vi "GetType.vi"(8 "error in (no error)":errorcluster, 11 "Load Pattern Msg":refnum<class "Load Pattern Msg.lvclass">) -> (0 "error out":errorcluster, 2 "Data Sample":variant, 3 "Load Pattern Msg":refnum<class "Load Pattern Msg.lvclass">)   [LabVIEW 2016, in "CS++PPG.lvlib" / "Load Pattern Msg.lvclass"]
uses:
  Load Pattern Msg.lvclass
  Load Pattern Msg.lvclass/Load Pattern Msg.ctl
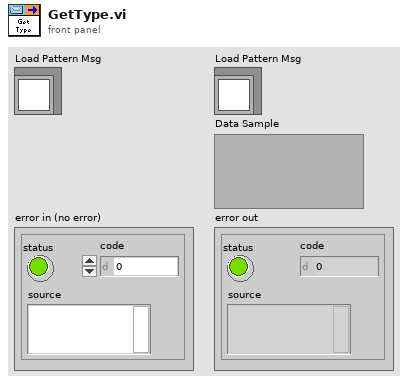
[diagram p1: front panel]
types:
  T1 = cluster{"TriggerCondition":i32, "TimeTable":dbl[], "ChannelTable":string[]}[]
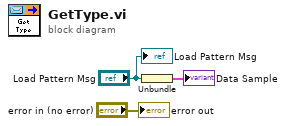
[diagram p0: block diagram]
diagram:
  n1 = Unbundle("Load Pattern Msg") -> (→"Data Sample":T1)
  "error out" <- "error in (no error)"
  "Load Pattern Msg" <- "Load Pattern Msg"
